vi "Filter.vi"(4 "Table":u16, 6 "Data":string[](array[string]), 7 "Filter In":T1[](array[typedef]), 8 "error in (no error)":errorcluster, 11 "Ref in":T3={"MS SQL Connection"=refnum, "UDL File"=path "", "Time"="", "DCODE"="", "WIP+1"=0, "MC No?"=0, "POKAYOKE?"=FALSE, "Expected Result"="", "Result [Status]"="", "Clock"=0.0, "RFID"="", "WIP Queue"=refnum, "TS Parameter"={"ProfitCenterCode"="", "LineCode"="", "WorkOrderNumber"="", "Model"="", "Model_with_Prefix"="", "VendorCode"="", "SetParameterDateCode"="", "PokaYoke"=0, "Target"=1, "Live_DateCode"="", "CustomerPartNumber"="", "Hand"="", "Ent_Stamp"=timestamp(0 s since 1904-01-01), "sBarcode"=FALSE, "FCA"=0, "STS_CD"=0.0}, "Data_Queue"=[], "RFID Serial No."=""} {"TS Parameter"."FCA" format="%01d"; "TS Parameter"."Target" min=1 max=100000; "TS Parameter"."PokaYoke" min=0 max=1}) -> (0 "error out":errorcluster, 5 "Filter Out":T1[](array[typedef]))   [LabVIEW 2020]
uses:
  Controls/TD SQL.ctl
  <vilib>/addons/database/Connection.llb/Conn ObjectReference.ctl
  Controls/WIP_State.ctl
  Controls/TS_Parameter.ctl
  Controls/Filter.ctl
  Controls/Comparator.ctl
  <vilib>/addons/database/NI_Database_API.lvlib
panel:
  in  "Apply":bool
  in  "OK Button":bool
  out "columns":string[](array[string])
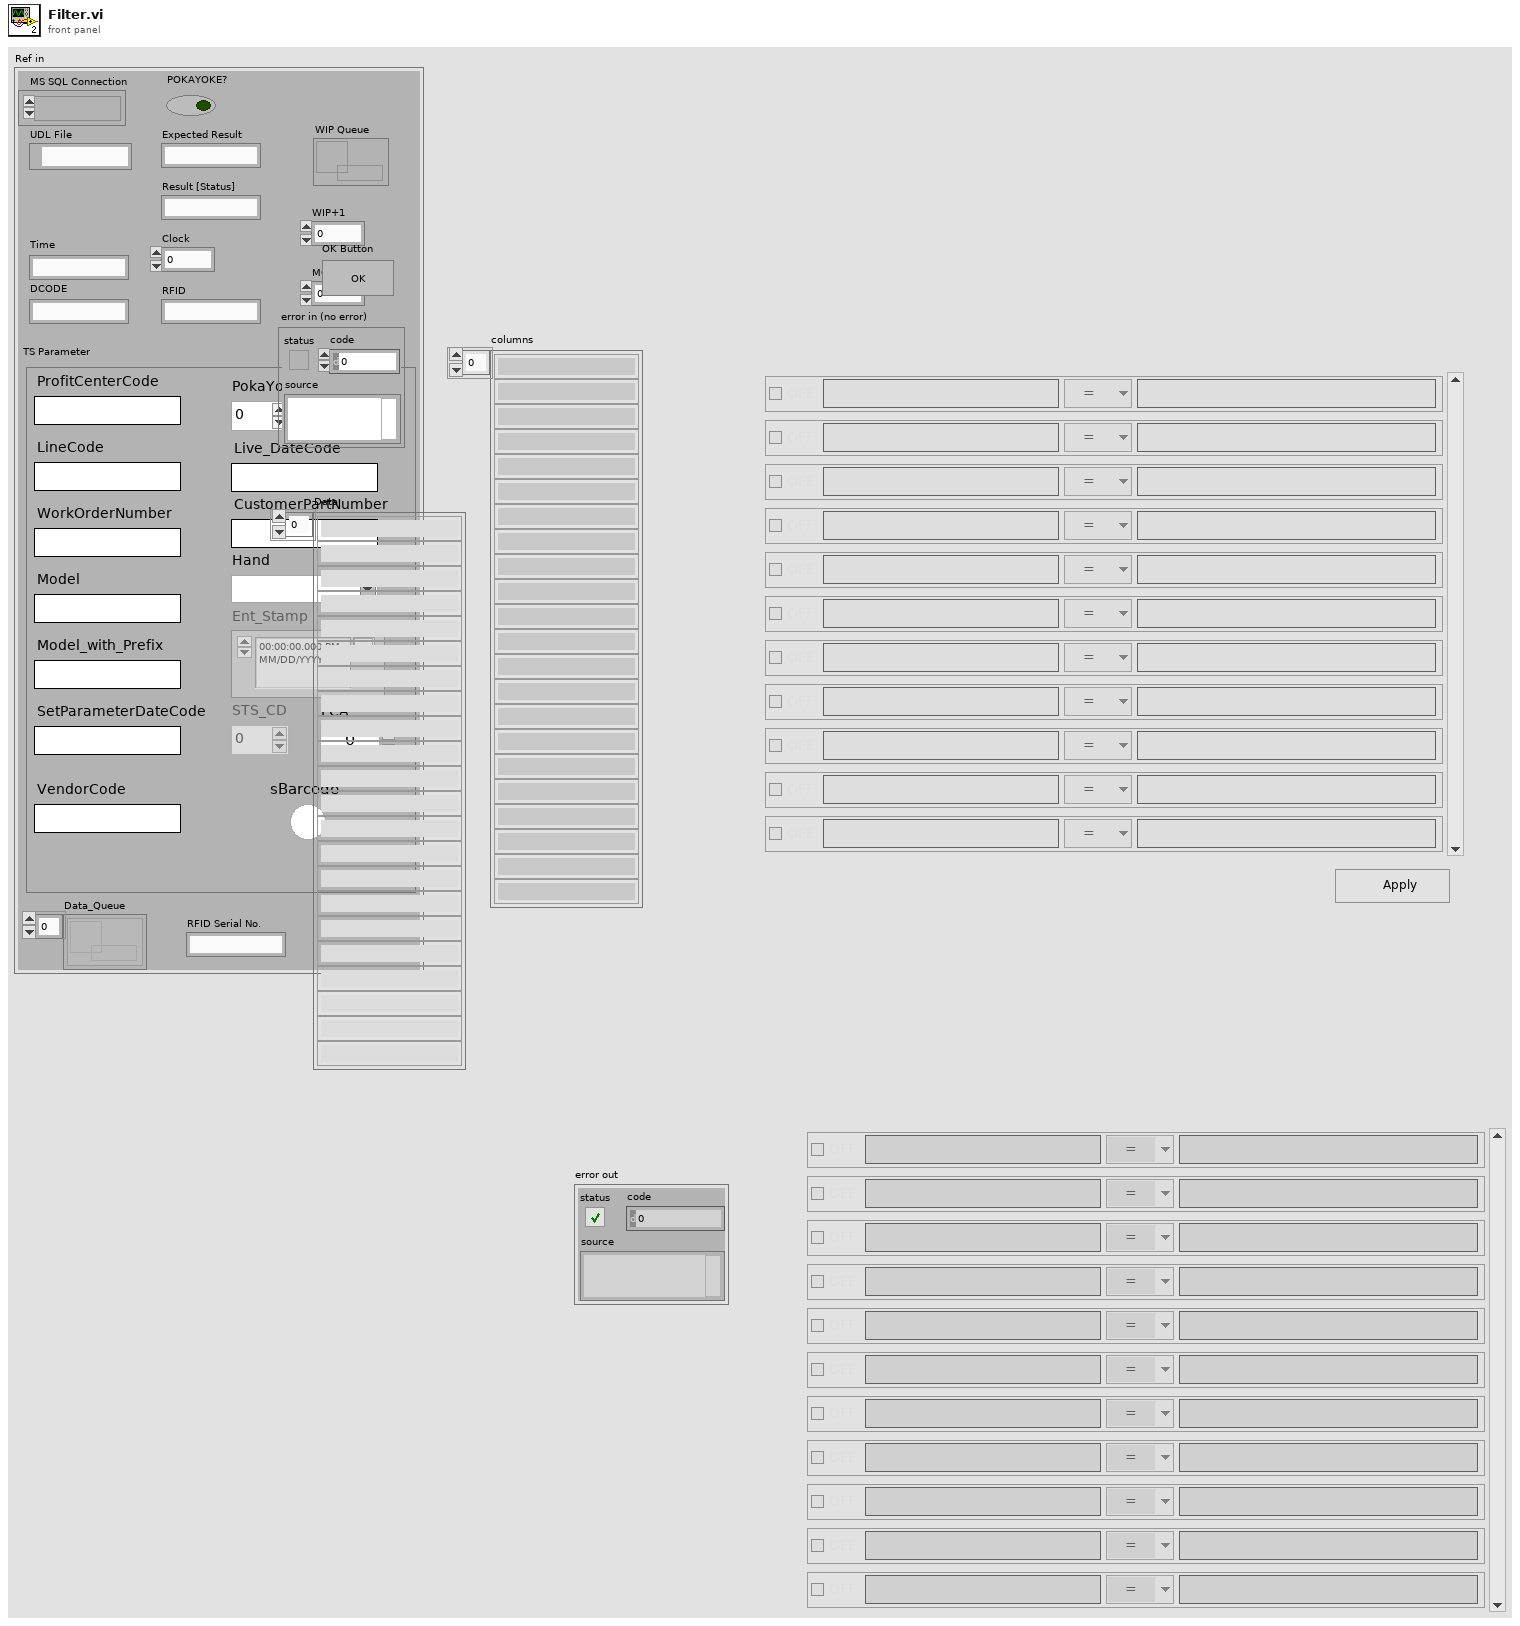
[diagram p1: front panel]
types:
  T1 = typedef "Filter.ctl" = cluster{"Select":bool, "Column":string, "Compare":T2, "Data":string}
  T2 = typedef "Comparator.ctl" = enum16{"=", "<=", ">=", "<", ">", "Like"}
  T3 = typedef "TD SQL.ctl" = cluster{"MS SQL Connection":T4, "UDL File":path, "Time":string, "DCODE":string, "WIP+1":i64, "MC No?":i32, "POKAYOKE?":bool, "Expected Result":string, "Result [Status]":string, "Clock":dbl, "RFID":string, "WIP Queue":refnum<queue>, "TS Parameter":T5, "Data_Queue":refnum<queue>[], "RFID Serial No.":string}
  T4 = typedef "NI_Database_API.lvlib/Conn ObjectReference.ctl" = refnum<k1>
  T5 = typedef "TS_Parameter.ctl" = cluster{"ProfitCenterCode":string, "LineCode":string, "WorkOrderNumber":string, "Model":string, "Model_with_Prefix":string, "VendorCode":string, "SetParameterDateCode":string, "PokaYoke":i32, "Target":i32, "Live_DateCode":string, "CustomerPartNumber":string, "Hand":string, "Ent_Stamp":timestamp, "sBarcode":bool, "FCA":i32, "STS_CD":dbl}
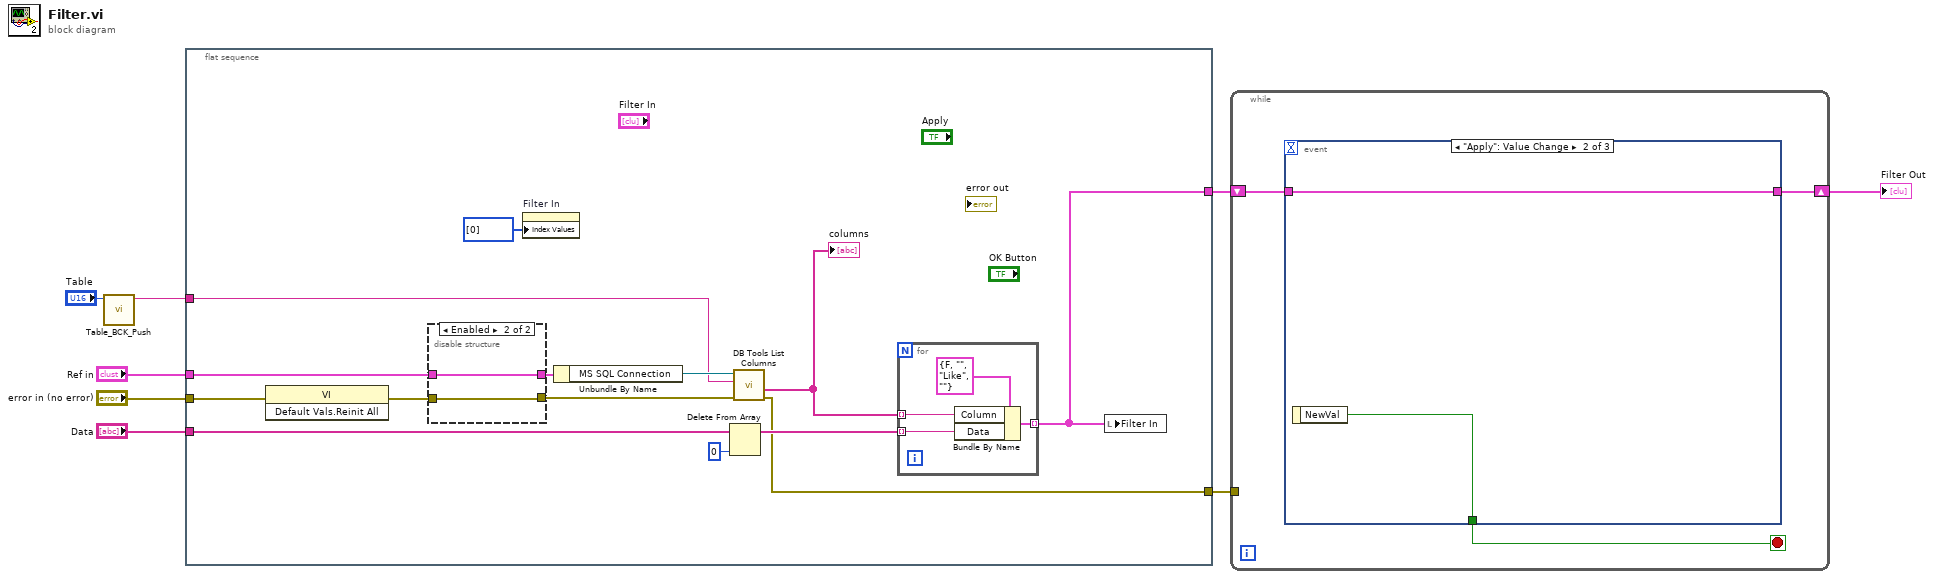
[diagram p0: block diagram]
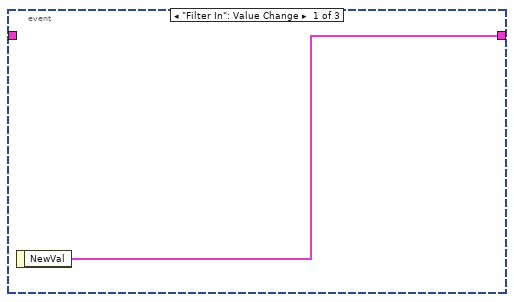
[diagram p2: hidden frame]
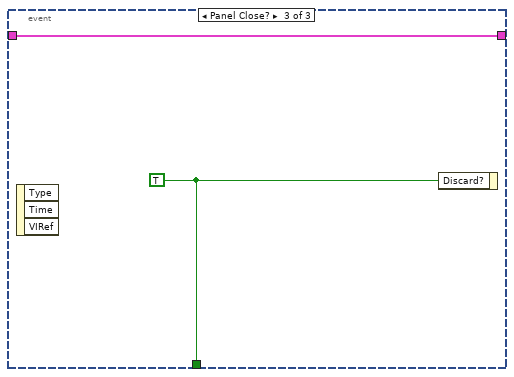
[diagram p3: hidden frame]
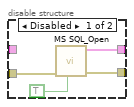
[diagram p4: hidden frame]
diagram:
  n1 = call "Table_BCK_Push.vi"("index"="Table") -> ("Table Name"=w2:string)  [unwired: 9 in, 1 out]
  n2 = flat-sequence {
    tunnel: [w16] -> w8
    tunnel: [w15] -> w7
    tunnel: "error in (no error)" -> [w11]
    tunnel: "Ref in" -> [w14]
    tunnel: w2 -> [w13]
    tunnel: "Data" -> [w12]
    frame #0 {
      n3 = invoke class="VI" method="Default Vals.Reinit All"(error in=w11) -> (error out=w10:errorcluster)  [unwired: 2 in, 2 out]
      n4 = disable-structure shown="Enabled" {
        disable-tunnel: w10 -> [w26 w27]
        disable-tunnel: [w25 w28] -> w22
        disable-tunnel: [w24 w27] -> w20
        disable-tunnel: w14 -> [_ w28]
        frame Disabled {
          n5 = call "MS SQL_Open.vi"("Bckup_DB?"=TRUE, "error in (no error)"=w26) -> ("error out"=w24:errorcluster, "Ref Out"=w25:T3)  [unwired: 7 in, 1 out]
        }
        frame Enabled {
        }
      }
      n6 = property on="Filter In" class="Arr (strict)"("Index Values"=u32[] [0]) -> ()  [unwired: 2 in, 2 out]
      n7 = Unbundle By Name(w22) -> ("MS SQL Connection"=w21:T4)
      n8 = Delete From Array(array=w12, index=0) -> (array with subset deleted=w18:string[])  [unwired: 1 in, 1 out]
      n9 = call <vilib>:"DB Tools List Columns.vi"("error in (no error)"=w20, "table"=w13, "connection reference"=w21) -> ("error out"=w16:errorcluster, "columns"=w19:string[])  [unwired: 1 in, 2 out]
      "columns" <- w19
      n10 = for {
        tunnel: w19 -> [w31] mode=indexing
        tunnel: [w30] -> w15 mode=indexing
        tunnel: w18 -> [w29] mode=indexing
        n11 = Bundle By Name(cluster=T1 {"Select"=FALSE, "Column"="", "Compare"=enum."Like", "Data"=""} ("Filter"), "Column"=w31, "Data"=w29) -> (w30:T1)
      }
      n12 = local write "Filter In"(w15) -> ()
    }
  }
  n13 = while {
    tunnel: w8 -> [_]
    shift-right: [w33] -> w6
    shift-left: w7 -> [w34]
    stop <- w35 stop-if-true
    n14 = event shown="[1] \"Apply\": Value Change" {
      selector: _ -> [_ _ _]
      dyn-events: _ -> [_ _ _]
      timeout: _ -> [_ _ _]
      tunnel: [_ w37 w40] -> w35
      tunnel: w34 -> [_ w38 w39]
      tunnel: [w36 w38 w39] -> w33
      event "Filter In": Value Change {
        n15 = event-data() -> ("NewVal"=w36:T1[])  [unwired: 1 in]
      }
      event "Apply": Value Change {
        n16 = event-data() -> ("NewVal"=w37:bool)  [unwired: 1 in]
      }
      event Panel Close? {
        w40 = TRUE ("Discard?")
        n17 = event-data() -> ()  [unwired: 1 in, 3 out]
        n18 = event-data("Discard?"=w40) -> ()  [unwired: 1 in, 1 out]
      }
    }
  }
  "Filter Out" <- w6
